vi "build_cmd.vi"(8 "error in (no error)":errorcluster, 9 "Parameter list":string[](array[string]), 10 "Command ID":string, 11 "Command class":string(combo)="G") -> (0 "error out":errorcluster, 2 "Command":string)   [LabVIEW 2018]
doc: "Start the active process or continue a process that is in the STOP state."
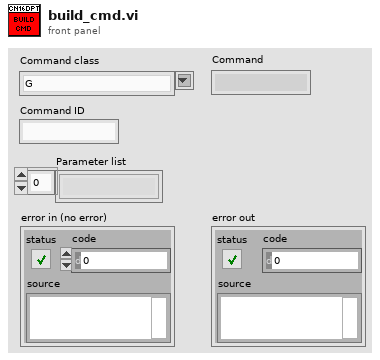
[diagram p1: front panel]
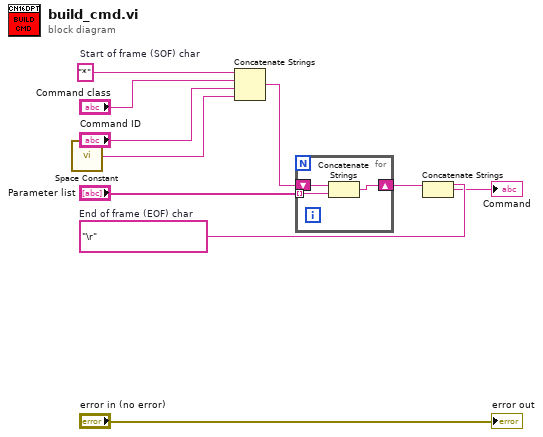
[diagram p0: block diagram]
diagram:
  w5 = "\r"  # End of frame (EOF) char
  w10 = "*"  # Start of frame (SOF) char
  n1 = call <vilib>:"Space Constant.vi"() -> ("String"=w7:string)
  n2 = Concatenate Strings(w10, "Command class", "Command ID", w7) -> (w3:string)
  n3 = for {
    shift-right: [w13] -> w6
    shift-left: w3 -> [w12]
    tunnel: "Parameter list" -> [w11] mode=indexing
    n4 = Concatenate Strings(w12, w11) -> (w13:string)
  }
  n5 = Concatenate Strings(w6, w5) -> (→"Command":string)
  "error out" <- "error in (no error)"
